vi "Telnet.vi"(7 "operaiton":T1, 8 "error in (no error)":errorcluster, 9 "CMD":string="/etc/init.d/qcmbr start", 10 "address":string="192.68.1.2", 11 "telnet connection in":T2) -> (0 "error out":errorcluster, 1 "data out":string, 2 "NeedRestart?":bool, 3 "telnet connection out":T2)   [LabVIEW 2015]
uses:
  <vilib>/addons/internet/telnet/telnet.llb/Telnet Session.ctl
  TelnetOperations.ctl
  <vilib>/addons/internet/NI_InternetTK_Core_VIs.lvlib
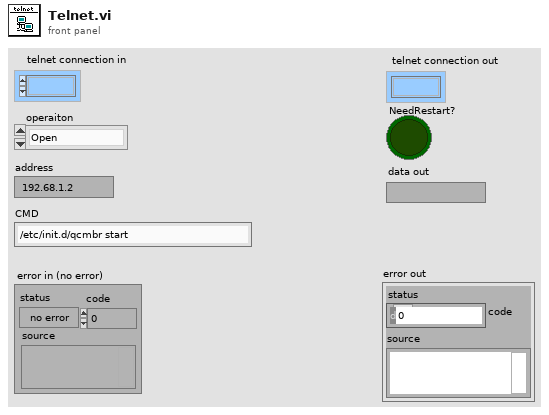
[diagram p1: front panel]
types:
  T1 = typedef "TelnetOperations.ctl" = enum16{"Open", "Write", "Read", "Start", "Restart", "Stop", "VerifyProcess", "Close"}
  T2 = typedef "Telnet Session.ctl" = refnum<k1>
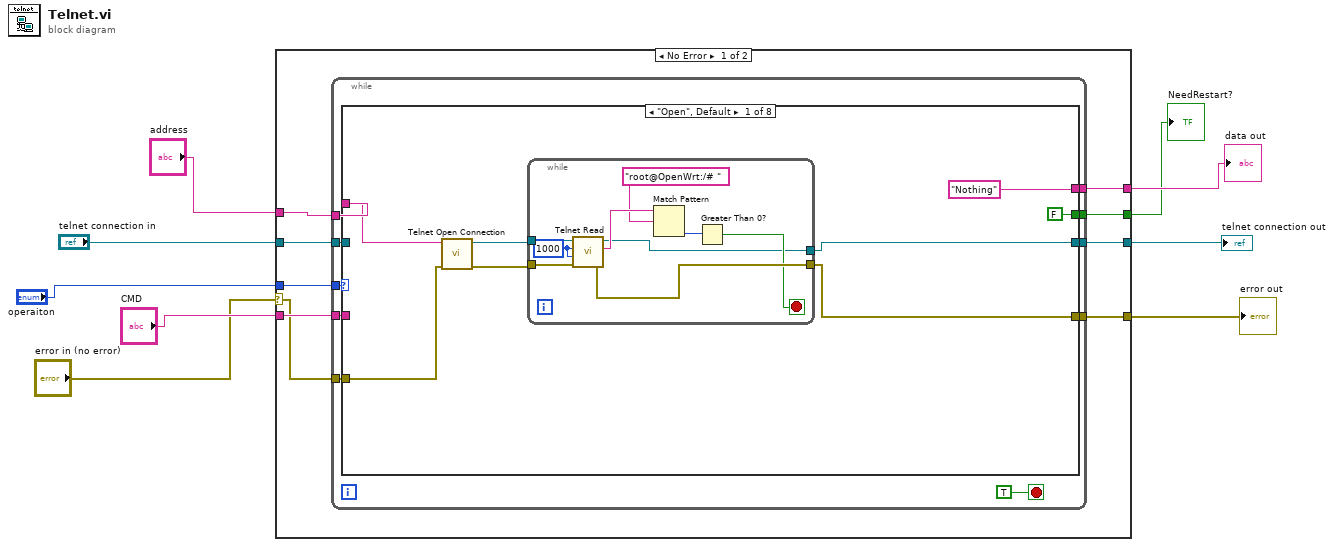
[diagram p0: block diagram]
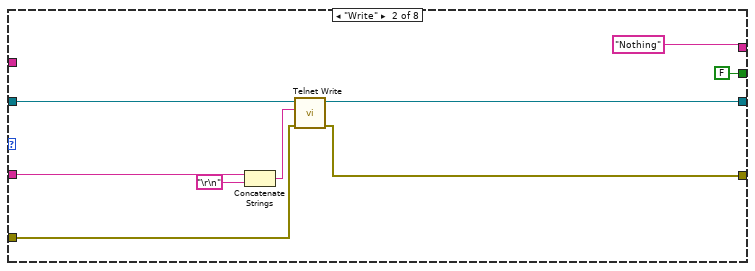
[diagram p2: hidden frame]
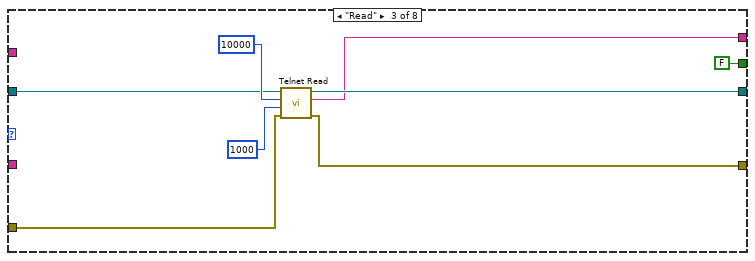
[diagram p3: hidden frame]
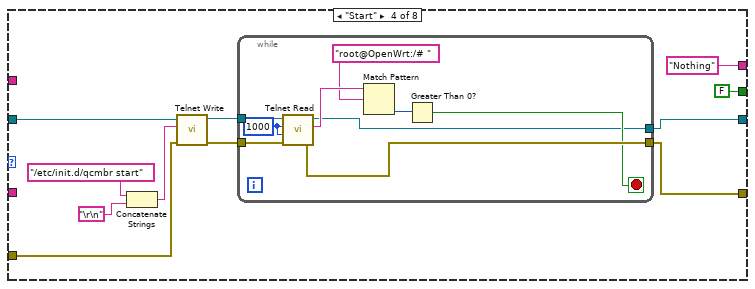
[diagram p4: hidden frame]
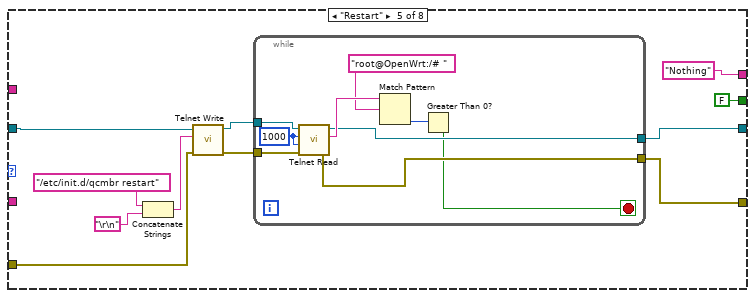
[diagram p5: hidden frame]
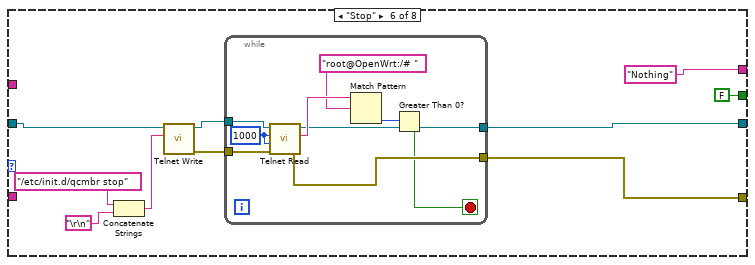
[diagram p6: hidden frame]
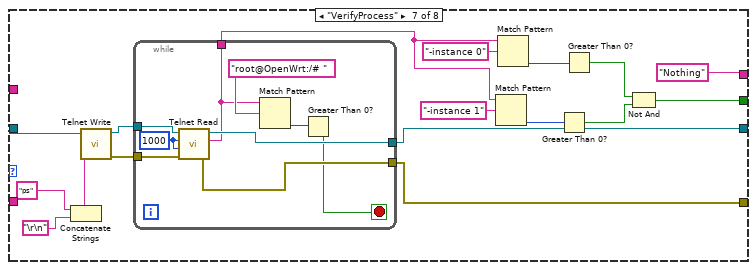
[diagram p7: hidden frame]
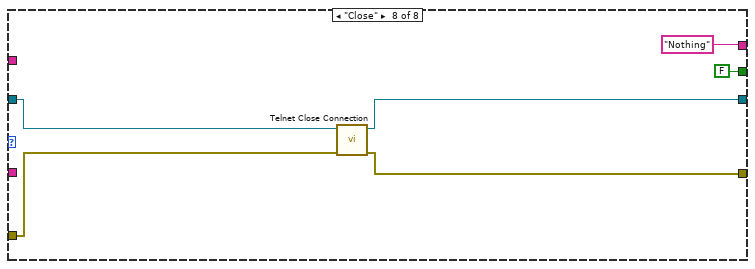
[diagram p8: hidden frame]
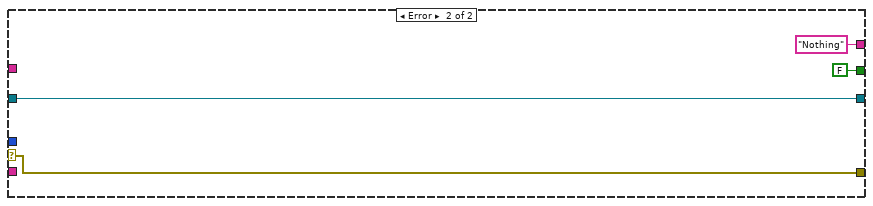
[diagram p9: hidden frame]
diagram:
  n1 = case shown="No Error" "error in (no error)" {
    selector: "error in (no error)" -> [w10 w154]
    tunnel: "operaiton" -> [w18 _]
    tunnel: "address" -> [w17 _]
    tunnel: [w16 w157] -> w7
    tunnel: "telnet connection in" -> [w15 w157]
    tunnel: [w14 "Nothing" ("data out")] -> w5
    tunnel: "CMD" -> [w13 _]
    tunnel: [w12 w154] -> w3
    tunnel: [w11 FALSE] -> w2
    frame No Error {
      n2 = while {
        tunnel: w18 -> [w27]
        tunnel: w17 -> [w26]
        tunnel: [w25] -> w16
        tunnel: w15 -> [w24]
        tunnel: [w23] -> w14
        tunnel: w13 -> [w22]
        tunnel: [w21] -> w12
        tunnel: w10 -> [w20]
        tunnel: [w19] -> w11
        stop <- TRUE stop-if-true
        n3 = case shown="\"Open\", Default" w27 {
          tunnel: w26 -> [w36 _ _ _ _ _ _ _]
          tunnel: [w34 w51 w60 w67 w89 w107 w132 w149] -> w25
          tunnel: w24 -> [_ w52 w59 w68 w90 w105 w133 w153]
          tunnel: ["Nothing" "Nothing" w58 "Nothing" "Nothing" "Nothing" "Nothing" "Nothing"] -> w23
          tunnel: w22 -> [_ w50 _ _ _ _ _ _]
          tunnel: [w32 w48 w56 w66 w88 w106 w131 w151] -> w21
          tunnel: w20 -> [w31 w49 w57 w65 w85 _ _ w152]
          tunnel: [FALSE FALSE FALSE FALSE FALSE FALSE w124 FALSE] -> w19
          frame "Open", Default {
            n4 = call <vilib>:"Telnet Open Connection.vi"("error in (no error)"=w31, "address"=w36) -> ("error out"=w33:errorcluster, "telnet connection"=w35:T2)  [unwired: 8 in]
            n5 = while {
              tunnel: w35 -> [w45]
              tunnel: [w37] -> w34
              tunnel: w33 -> [w44]
              tunnel: [w43] -> w32
              stop <- w39 stop-if-true
              w38 = 1000 ("bytes to read")
              n6 = call <vilib>:"Telnet Read.vi"("error in (no error)"=w44, "timeout ms (25000)"=w38, "bytes to read"=w38, "telnet connection"=w45) -> ("error out"=w43:errorcluster, "data out"=w42:string, "telnet connection out"=w37:T2)  [unwired: 3 in]
              n7 = Match Pattern(string=w42, regular expression="root@OpenWrt:/# ") -> (offset past match=w40:i32)  [unwired: 1 in, 3 out]
              n8 = Greater Than 0?(x=w40) -> (x > 0?=w39:bool)
            }
          }
          frame "Write" {
            n9 = Concatenate Strings(w50, "\r\n") -> (w53:string)
            n10 = call <vilib>:"Telnet Write.vi"("error in (no error)"=w49, "data in"=w53, "telnet connection"=w52) -> ("error out"=w48:errorcluster, "telnet connection out"=w51:T2)  [unwired: 4 in, 1 out]
          }
          frame "Read" {
            n11 = call <vilib>:"Telnet Read.vi"("error in (no error)"=w57, "timeout ms (25000)"=1000, "bytes to read"=10000, "telnet connection"=w59) -> ("error out"=w56:errorcluster, "data out"=w58:string, "telnet connection out"=w60:T2)  [unwired: 3 in]
          }
          frame "Start" {
            n12 = Concatenate Strings("/etc/init.d/qcmbr start" ("data in"), "\r\n") -> (w69:string)
            n13 = call <vilib>:"Telnet Write.vi"("error in (no error)"=w65, "data in"=w69, "telnet connection"=w68) -> ("error out"=w72:errorcluster, "telnet connection out"=w73:T2)  [unwired: 4 in, 1 out]
            n14 = while {
              tunnel: w73 -> [w82]
              tunnel: [w74] -> w67
              tunnel: w72 -> [w81]
              tunnel: [w80] -> w66
              stop <- w76 stop-if-true
              w75 = 1000 ("bytes to read")
              n15 = call <vilib>:"Telnet Read.vi"("error in (no error)"=w81, "timeout ms (25000)"=w75, "bytes to read"=w75, "telnet connection"=w82) -> ("error out"=w80:errorcluster, "data out"=w79:string, "telnet connection out"=w74:T2)  [unwired: 3 in]
              n16 = Match Pattern(string=w79, regular expression="root@OpenWrt:/# ") -> (offset past match=w77:i32)  [unwired: 1 in, 3 out]
              n17 = Greater Than 0?(x=w77) -> (x > 0?=w76:bool)
            }
          }
          frame "Restart" {
            n18 = Concatenate Strings("/etc/init.d/qcmbr restart" ("data in"), "\r\n") -> (w91:string)
            n19 = call <vilib>:"Telnet Write.vi"("error in (no error)"=w85, "data in"=w91, "telnet connection"=w90) -> ("error out"=w87:errorcluster, "telnet connection out"=w86:T2)  [unwired: 4 in, 1 out]
            n20 = while {
              tunnel: [w98] -> w89
              tunnel: [w97] -> w88
              tunnel: w87 -> [w95]
              tunnel: w86 -> [w94]
              stop <- w96 stop-if-true
              w99 = 1000 ("bytes to read")
              n21 = call <vilib>:"Telnet Read.vi"("error in (no error)"=w95, "timeout ms (25000)"=w99, "bytes to read"=w99, "telnet connection"=w94) -> ("error out"=w97:errorcluster, "data out"=w102:string, "telnet connection out"=w98:T2)  [unwired: 3 in]
              n22 = Match Pattern(string=w102, regular expression="root@OpenWrt:/# ") -> (offset past match=w100:i32)  [unwired: 1 in, 3 out]
              n23 = Greater Than 0?(x=w100) -> (x > 0?=w96:bool)
            }
          }
          frame "Stop" {
            n24 = Concatenate Strings("/etc/init.d/qcmbr stop" ("data in"), "\r\n") -> (w110:string)
            n25 = call <vilib>:"Telnet Write.vi"("data in"=w110, "telnet connection"=w105) -> ("error out"=w109:errorcluster, "telnet connection out"=w108:T2)  [unwired: 5 in, 1 out]
            n26 = while {
              tunnel: [w117] -> w107
              tunnel: [w116] -> w106
              tunnel: w109 -> [w114]
              tunnel: w108 -> [w113]
              stop <- w115 stop-if-true
              w118 = 1000 ("bytes to read")
              n27 = call <vilib>:"Telnet Read.vi"("error in (no error)"=w114, "timeout ms (25000)"=w118, "bytes to read"=w118, "telnet connection"=w113) -> ("error out"=w116:errorcluster, "data out"=w121:string, "telnet connection out"=w117:T2)  [unwired: 3 in]
              n28 = Match Pattern(string=w121, regular expression="root@OpenWrt:/# ") -> (offset past match=w119:i32)  [unwired: 1 in, 3 out]
              n29 = Greater Than 0?(x=w119) -> (x > 0?=w115:bool)
            }
          }
          frame "VerifyProcess" {
            n30 = Concatenate Strings("ps" ("data in"), "\r\n") -> (w136:string)
            n31 = call <vilib>:"Telnet Write.vi"("data in"=w136, "telnet connection"=w133) -> ("error out"=w135:errorcluster, "telnet connection out"=w134:T2)  [unwired: 5 in, 1 out]
            n32 = while {
              tunnel: [w144] -> w132
              tunnel: [w143] -> w131
              tunnel: w135 -> [w141]
              tunnel: w134 -> [w140]
              tunnel: [w139] -> w123
              stop <- w142 stop-if-true
              w145 = 1000 ("bytes to read")
              n33 = call <vilib>:"Telnet Read.vi"("error in (no error)"=w141, "timeout ms (25000)"=w145, "bytes to read"=w145, "telnet connection"=w140) -> ("error out"=w143:errorcluster, "data out"=w139:string, "telnet connection out"=w144:T2)  [unwired: 3 in]
              n34 = Match Pattern(string=w139, regular expression="root@OpenWrt:/# ") -> (offset past match=w146:i32)  [unwired: 1 in, 3 out]
              n35 = Greater Than 0?(x=w146) -> (x > 0?=w142:bool)
            }
            n36 = Match Pattern(string=w123, regular expression="-instance 1") -> (offset past match=w128:i32)  [unwired: 1 in, 3 out]
            n37 = Match Pattern(string=w123, regular expression="-instance 0") -> (offset past match=w127:i32)  [unwired: 1 in, 3 out]
            n38 = Greater Than 0?(x=w128) -> (x > 0?=w125:bool)
            n39 = Greater Than 0?(x=w127) -> (x > 0?=w126:bool)
            n40 = Not And(1:w125, 2:w126) -> (0:w124:bool)
          }
          frame "Close" {
            n41 = call <vilib>:"Telnet Close Connection.vi"("error in (no error)"=w152, "telnet connection"=w153) -> ("error out"=w151:errorcluster, "telnet connection out"=w149:T2)  [unwired: 8 in]
          }
        }
      }
    }
    frame Error {
    }
  }
  "telnet connection out" <- w7
  "data out" <- w5
  "error out" <- w3
  "NeedRestart?" <- w2
